vi "Read Waveform (DBL).vi"(8 "error in (no error)":errorcluster, 11 "Async Data in":T1) -> (0 "error out":errorcluster, 1 "Properties":T4={"Data reference"=0, "t0 at start"=timestamp(0 s since 1904-01-01), "dt"=nan, "offset from start (samples)"=0}, 2 "Data":dbl[](array[numeric]), 3 "Received Wfm":refnum<data-value>, 4 "Receive Time":timestamp, 5 "Async Data out":T1)   [LabVIEW 2012, in "Waveform Data Logger Engine.lvlib"]
uses:
  Waveform Data Logger Engine.lvlib
  Types/Async Data.ctl
  Classes/Waveforms/Utilities/Reference Dictionary/Reference Dictionary.lvclass
  <vilib>/NI Veristand/Custom Device Waveform API/Multiple Waveforms Read (DBL)/Multiple Waveforms Read (DBL).lvclass
  Types/Wfm Acq Data.ctl
  Classes/Waveforms/Waveform Receive/Waveform Receive.lvclass
  Classes/Waveforms/Waveform Log/Waveform Log.lvclass
  Types/Async Communication.ctl
  Types/Check File Loop Cmd.ctl
  <vilib>/NI Veristand/Custom Device Waveform API/Waveform properties.ctl
  <vilib>/NI Veristand/Custom Device API/Waveform Data Reference.ctl
  <vilib>/NI Veristand/Custom Device Waveform API/Waveform Session.lvclass/Waveform Session.ctl
  <vilib>/NI Veristand/Custom Device Waveform API/Multiple Waveforms Read (DBL)/Multiple Waveforms Read (DBL).lvclass/Multiple Waveforms Read (DBL).ctl
  <vilib>/NI Veristand/Custom Device Waveform API/Internal Comm Classes/WPL Comm/WPL Comm (1D DBL)/WPL Comm (1D DBL).lvclass/WPL Comm (1D DBL).ctl
  Classes/Waveforms/Utilities/Reference Dictionary/Reference Dictionary.lvclass/Reference Dictionary.ctl
  <vilib>/NI Veristand/Custom Device Waveform API/Multiple Waveforms Read (DBL)/NI VeriStand - Read Multiple Waveforms (DBL).vi
  <vilib>/NI Veristand/Custom Device Waveform API/Internal Comm Classes/WPL Comm/WPL Comm (1D DBL)/Comm_read 1d dbl.vi
  <vilib>/NI Veristand/Custom Device Waveform API/Check Opened.vi
  <vilib>/NI Veristand/Custom Device Waveform API/Internal Comm Classes/WPL Comm/Convert Q Error to Shutdown Error.vi
  <vilib>/Utility/error.llb/Error Cluster From Error Code.vi
  <vilib>/NI VeriStand/Custom Device Waveform API/NI_VS Custom Device Waveform API.lvlib
  <vilib>/NI VeriStand/Custom Device API/Custom Device API.lvlib
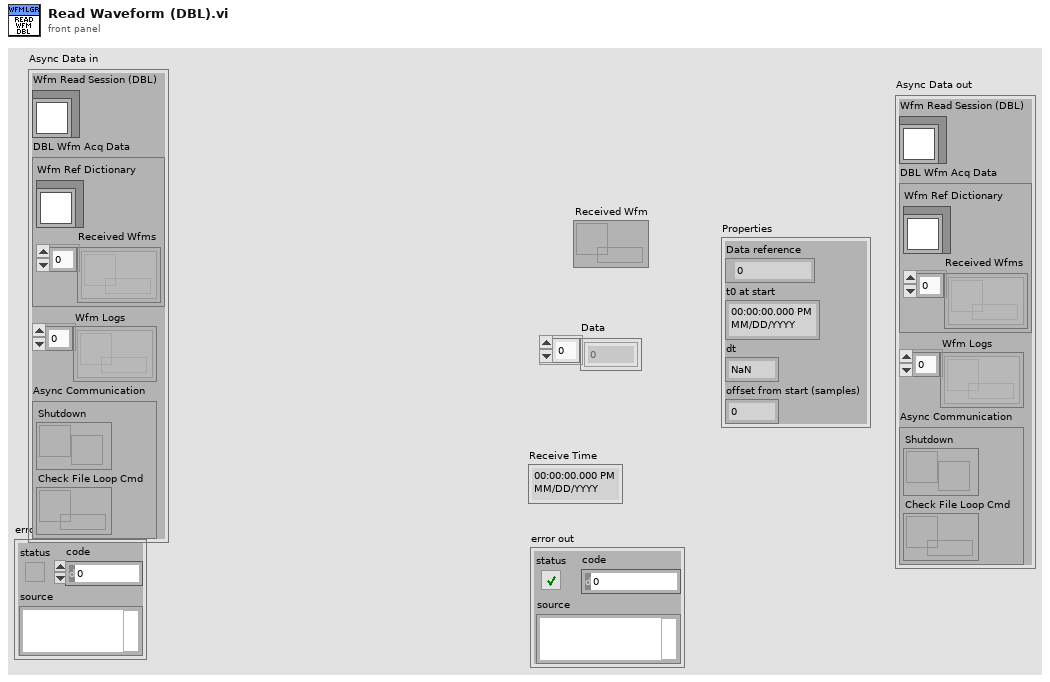
[diagram p1: front panel]
types:
  T1 = typedef "Waveform Data Logger Engine.lvlib/Async Data.ctl" = cluster{"Wfm Read Session (DBL)":refnum<class "Multiple Waveforms Read (DBL).lvclass">, "DBL Wfm Acq Data":T2, "Wfm Logs":refnum<data-value>[], "Async Communication":T3}
  T2 = typedef "Waveform Data Logger Engine.lvlib/Wfm Acq Data.ctl" = cluster{"Wfm Ref Dictionary":refnum<class "Reference Dictionary.lvclass">, "Received Wfms":refnum<data-value>[]}
  T3 = typedef "Waveform Data Logger Engine.lvlib/Async Communication.ctl" = cluster{"Shutdown":refnum<user-event>, "Check File Loop Cmd":refnum<queue>}
  T4 = typedef "NI_VS Custom Device Waveform API.lvlib/Waveform properties.ctl" = cluster{"Data reference":T5, "t0 at start":timestamp, "dt":dbl, "offset from start (samples)":u64}
  T5 = typedef "Custom Device API.lvlib/Waveform Data Reference.ctl" = i32
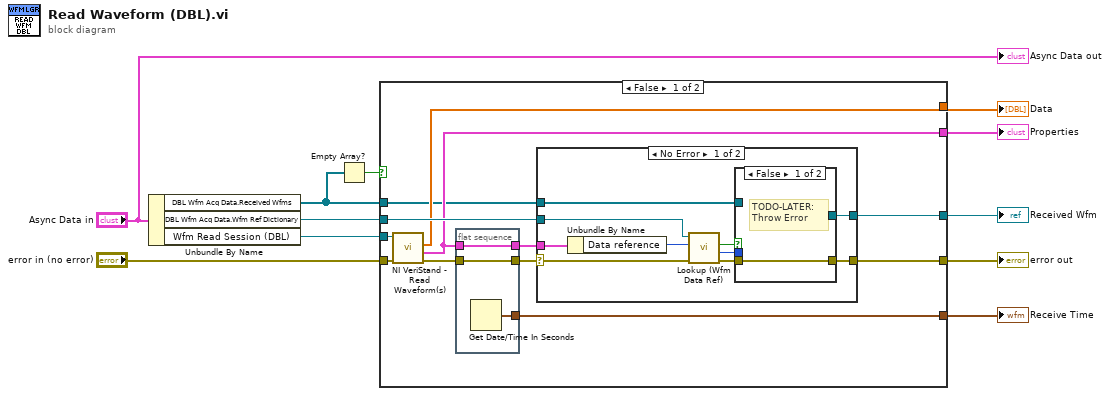
[diagram p0: block diagram]
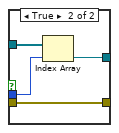
[diagram p2: hidden frame]
diagram:
  n1 = Unbundle By Name("Async Data in") -> ("DBL Wfm Acq Data.Received Wfms"=w2:refnum<data-value>[], "DBL Wfm Acq Data.Wfm Ref Dictionary"=w8:refnum<class "Reference Dictionary.lvclass">, "Wfm Read Session (DBL)"=w9:refnum<class "Multiple Waveforms Read (DBL).lvclass">)
  n2 = Empty Array?(array=w2) -> (empty?=w1:bool)
  n3 = case shown="False" w1 {
    tunnel: "error in (no error)" -> [w23 w43]
    tunnel: [w22 w43] -> w10
    tunnel: w9 -> [w21 _]
    tunnel: w8 -> [w20 _]
    tunnel: [w19 _] -> w7
    tunnel: [w16 _] -> w6
    tunnel: [w15 _] -> w5
    tunnel: [w13 _] -> w4
    tunnel: w2 -> [w12 _]
    frame False {
      n4 = call-poly <vilib>:"NI VeriStand - Read Waveform(s).vi"("error in (no error)"=w23, "Multiple Waveforms Read Session (DBL) in"=w21) -> ("error out"=w18:errorcluster, "Properties"=w13:T4, "Data"=w19:dbl[])  [unwired: 5 in, 2 out]
      n5 = flat-sequence {
        tunnel: w18 -> [w26]
        tunnel: [w26] -> w17
        tunnel: [w25] -> w15
        tunnel: [w24] -> w14
        tunnel: w13 -> [w24]
        frame #0 {
          n6 = Get Date/Time In Seconds() -> (seconds since 1Jan1904=w25:timestamp)
        }
      }
      n7 = case shown="No Error" w17 {
        selector: w17 -> [w31 w42]
        tunnel: w14 -> [w27 _]
        tunnel: [w33 w42] -> w22
        tunnel: w20 -> [w32 _]
        tunnel: w12 -> [w29 _]
        tunnel: [w28 _] -> w16
        frame No Error {
          n8 = Unbundle By Name(w27) -> ("Data reference"=w36:T5)
          n9 = call "Lookup (Wfm Data Ref).vi"("error in (no error)"=w31, "Wfm Data Ref"=w36, "Reference Dictionary in"=w32) -> ("error out"=w34:errorcluster, "Index"=w30:i32, "Found"=w35:bool)  [unwired: 5 in, 1 out]
          n10 = case shown="False" w35 {
            tunnel: w34 -> [w37 w38]
            tunnel: [w37 w38] -> w33
            tunnel: w30 -> [_ w41]
            tunnel: w29 -> [_ w40]
            tunnel: [_ w39] -> w28
            frame False {
              # "TODO-LATER:\nThrow Error"
            }
            frame True {
              n11 = Index Array(array=w40, index=w41) -> (element=w39:refnum<data-value>)
            }
          }
        }
        frame Error {
        }
      }
    }
    frame True {
    }
  }
  "error out" <- w10
  "Data" <- w7
  "Received Wfm" <- w6
  "Properties" <- w4
  "Receive Time" <- w5
  "Async Data out" <- "Async Data in"
